vi "test btn dialog with tmo.vi"() -> ()   [LabVIEW 2017]
panel:
  out "true":bool
  out "T button?":bool
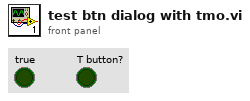
[diagram p1: front panel]
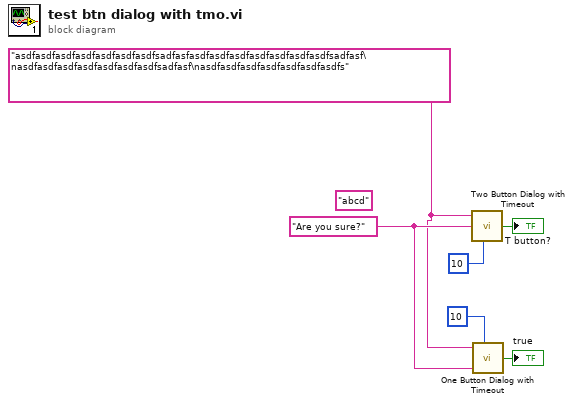
[diagram p0: block diagram]
diagram:
  (unwired) "abcd" ("Text")
  w1 = "asdfasdfasdfasdfasdfasdfasdfsadfasfasdfasdfasdfasdfasdfasdfasdfsadfasf\nasdfasdfasdfasdfasdfasdfasdfsadfasf\nasdfasdfasdfasdfasdfasdfasdfs" ("Text")
  w2 = "Are you sure?" ("T button name (\"OK\")")
  n1 = call "Two Button Dialog with Timeout.vi"("message"=w1, "T button name (\"OK\")"=w2, "F Timeout(-1 s)"=10 ("T Timeout(-1 s)")) -> ("T button?"=→"T button?":bool)  [unwired: 6 in]
  n2 = call "One Button Dialog with Timeout.vi"("message"=w1, "Btn Timeout(-1 s)"=10, "T button name (\"OK\")"=w2) -> ("true"=→"true":bool)  [unwired: 6 in]
